vi "VI Clipboard Paste.vi"(8 "error in (no error)":errorcluster, 10 "Drop Position (0, 0)":cluster{"Left":i32, "Top":i32}, 11 "VI Refnum in":refnum<vi>) -> (0 "error out":errorcluster, 3 "VI Refnum out":refnum<vi>)   [LabVIEW 2022 SP3, in "VI-Snippet.lvlib"]
doc: "Pastes the clipboard content into the <b>VI Refnum in</b> block diagram. Specify the <b>Drop Position</b> where the objects should be positioned relative to the current diagram window origin."
uses:
  VI-Snippet.lvlib
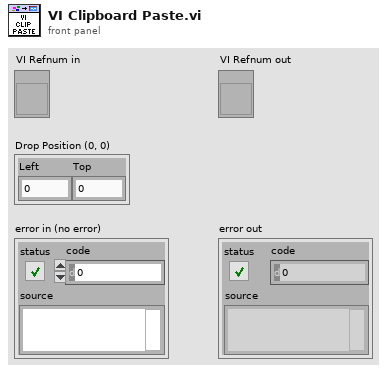
[diagram p1: front panel]
types:
  T1 = typedef "LVPointTypeDef.ctl" = cluster{"Horizontal":i16, "Vertical":i16}
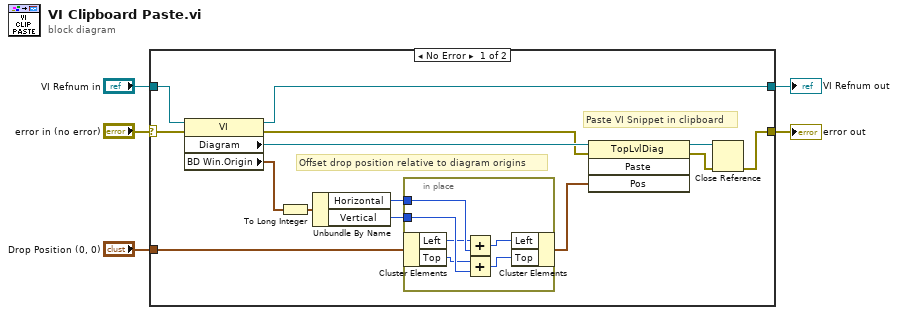
[diagram p0: block diagram]
diagram:
  n1 = case shown="No Error" "error in (no error)" {
    selector: "error in (no error)" -> [w6 w27]
    tunnel: "VI Refnum in" -> [w19 w26]
    tunnel: "Drop Position (0, 0)" -> [w18 _]
    tunnel: [w17 w27] -> w3
    tunnel: [w16 w26] -> w1
    frame No Error {
      # "Paste VI Snippet in clipboard"
      # "Offset drop position relative to diagram origins"
      n2 = property class="VI"(reference=w19, error in=w6) -> (reference out=w16:refnum<vi>, error out=w12:errorcluster, "Diagram"=w13:refnum<vi>, "BD Win.Origin"=w11:T1)
      n3 = To Long Integer(number=w11) -> (32bit integer=w7:cluster{"Horizontal":i32, "Vertical":i32})
      n4 = Unbundle By Name(w7) -> ("Horizontal"=w10:i32, "Vertical"=w9:i32)
      n5 = in-place {
        in-place-border: w10 -> [w25]
        in-place-border: w9 -> [w24]
        n6 = in-place-cluster #1(w18) -> ("Left"=w23:i32, "Top"=w22:i32)
        n7 = Add(x=w23, y=w25) -> (x+y=w21:i32)
        n8 = Add(x=w22, y=w24) -> (x+y=w20:i32)
        n9 = in-place-cluster #1("Left"=w21, "Top"=w20) -> (w8:cluster{"Left":i32, "Top":i32})
      }
      n10 = invoke class="TopLvlDiag" method="Paste"(reference=w13, error in=w12, "Pos"=w8) -> (reference out=w15:refnum<vi>, error out=w14:errorcluster)  [unwired: 1 in, 2 out]
      n11 = Close Reference(reference=w15, error in (no error)=w14) -> (error out=w17:errorcluster)
    }
    frame Error {
    }
  }
  "error out" <- w3
  "VI Refnum out" <- w1
